vi "C37 UTIL Clean Closing Sign from Pointer String.vi"(11 "String In":string) -> (3 "String Out":string)   [LabVIEW 2013, in "C37118-DLL.lvlib"]
uses:
  C37118-DLL.lvlib
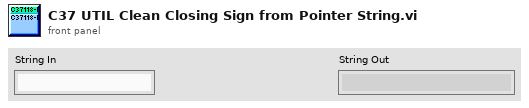
[diagram p1: front panel]
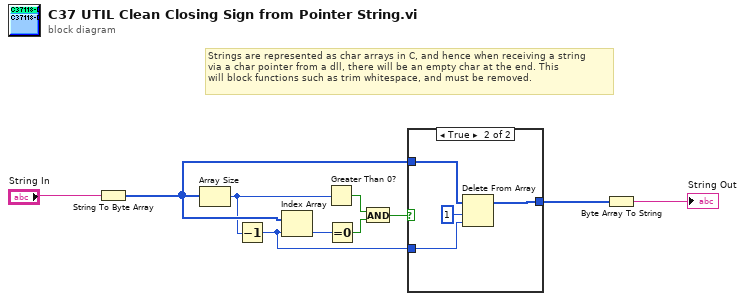
[diagram p0: block diagram]
diagram:
  # "Strings are represented as char arrays in C, and hence when receiving a string\nvia a char pointer from a dll, there will be an empty char at the end. This\nwill block functions such as trim whitespace, and must be removed."
  n1 = String To Byte Array(string="String In") -> (unsigned byte array=w4:u8[])
  n2 = Array Size(array=w4) -> (size(s)=w3:i32)
  n3 = Decrement(x=w3) -> (x-1=w8:i32)
  n4 = Index Array(array=w4, index=w8) -> (element=w2:u8)
  n5 = Greater Than 0?(x=w3) -> (x > 0?=w6:bool)
  n6 = Equal To 0?(x=w2) -> (x = 0?=w5:bool)
  n7 = And(x=w6, y=w5) -> (x .and. y?=w7:bool)
  n8 = case shown="True" w7 {
    tunnel: w4 -> [w11 w15]
    tunnel: w8 -> [_ w14]
    tunnel: [w11 w12] -> w9
    frame False {
    }
    frame True {
      n9 = Delete From Array(array=w15, length=1, index=w14) -> (array with subset deleted=w12:u8[])  [unwired: 1 out]
    }
  }
  n10 = Byte Array To String(unsigned byte array=w9) -> (string=→"String Out":string)
